vi "Actor Core.vi"(8 "error in":errorcluster, 11 "SpectrometerUI in":refnum<class "SpectrometerUI.lvclass">) -> (0 "error out":errorcluster, 3 "Actor out":refnum<class "Actor.lvclass">)   [LabVIEW 2023, in "SpectrometerUI.lvlib" / "SpectrometerUI.lvclass"]
doc: "(<B>Filename</B>: Actor Framework.lvlib:Actor.lvclass:Actor Core.vi)\n\nReceives messages to the actor, reacts to them, and initiates any error handling that may shut the actor down.\n\nDescendant classes may override this VI to append parallel tasks for the actor to complete while it handles messages. Overrides use the Call Parent Class Method node."
uses:
  SpectrometerUI.lvclass
  C:/Program Files/National Instruments/LabVIEW 2023/vi.lib/ActorFramework/Actor/Actor.lvclass
  <vilib>/ActorFramework/Actor/Actor.lvclass
  <vilib>/ActorFramework/Message Enqueuer/Message Enqueuer.lvclass
  typedefs/SpectroData.ctl
  ConcreteClasses/ConcreteInstrumentClasses/SpectrometerClasses/Spectrometer_HRS_LV/HRS_Spectrometer/HRS_Spectrometer/HRS_Spectrometer.lvclass
  <vilib>/ActorFramework/Actor/Actor.lvclass/Actor.ctl
  <vilib>/ActorFramework/Message Enqueuer/Message Enqueuer.lvclass/Message Enqueuer.ctl
  SpectrometerUI.lvclass/SpectrometerUI.ctl
  Interfaces/InitDeinitInterface/InitDeinit Messages/Init Msg/Init Msg.lvclass/Init Msg.ctl
  Interfaces/AbstractInstrumentClasses/Spectrometers_LV/Spectrometer Messages/GoToWavelength Msg/GoToWavelength Msg.lvclass/GoToWavelength Msg.ctl
  Interfaces/AbstractInstrumentClasses/Spectrometers_LV/Spectrometer Messages/SetMirror Msg/SetMirror Msg.lvclass/SetMirror Msg.ctl
  Interfaces/AbstractInstrumentClasses/Spectrometers_LV/Spectrometer Messages/SetSlitwidth Msg/SetSlitwidth Msg.lvclass/SetSlitwidth Msg.ctl
  Interfaces/AbstractInstrumentClasses/Spectrometers_LV/Spectrometer Messages/ChangeGrating Msg/ChangeGrating Msg.lvclass/ChangeGrating Msg.ctl
  <vilib>/ActorFramework/Message Enqueuer/Init from Existing Queue.vi
  <vilib>/ActorFramework/Message Enqueuer/Enqueue.vi
  Interfaces/InitDeinitInterface/InitDeinit Messages/DeInit Msg/DeInit Msg.lvclass
  C:/Program Files/National Instruments/LabVIEW 2023/vi.lib/ActorFramework/Message/Message.lvclass
  Interfaces/InitDeinitInterface/InitDeinit Messages/Init Msg/Init Msg.lvclass
  Interfaces/AbstractInstrumentClasses/Spectrometers_LV/Spectrometer Messages/GoToWavelength Msg/GoToWavelength Msg.lvclass
  Interfaces/AbstractInstrumentClasses/Spectrometers_LV/Spectrometer Messages/SetMirror Msg/SetMirror Msg.lvclass
  <vilib>/ActorFramework/Stop Msg/Stop Msg.lvclass
  Interfaces/AbstractInstrumentClasses/Spectrometers_LV/Spectrometer Messages/SetSlitwidth Msg/SetSlitwidth Msg.lvclass
  Interfaces/AbstractInstrumentClasses/Spectrometers_LV/Spectrometer Messages/ChangeGrating Msg/ChangeGrating Msg.lvclass
  <vilib>/ActorFramework/Message Priority Queue/Priority Enqueue.vi
  SpectrometerUI.lvlib
  typedefs/typedefs.lvlib
panel:
  out "Self Enqueuer":refnum<class "Message Enqueuer.lvclass">
  in  "stop":bool
  in  "Set FrEnt Slitwidth":bool
  in  "Front Entrance":dbl
  in  "Set SidEnt Slitwidth":bool
  in  "Side Entrance":dbl
  in  "Set FrExSlitwidth":bool
  in  "Front Exit":dbl
  in  "Exit":enum16{"FRONT", "SIDE"}(ring)
  in  "Entrance":enum16{"FRONT", "SIDE"}(ring)
  in  "SpectroCluster":T1
  out "HRS Enqueuer":refnum<class "Message Enqueuer.lvclass">
  in  "Set Grating":bool
  in  "Grating":u8=1 min=1 max=3
  in  "Set Wavelength":bool
  in  "Wavelength":dbl
  in  "Set SidExSlitwidth":bool
  in  "Side Exit":dbl
  in  "Connect":bool
  in  "VISA resource name":refnum<visa-resource-name>
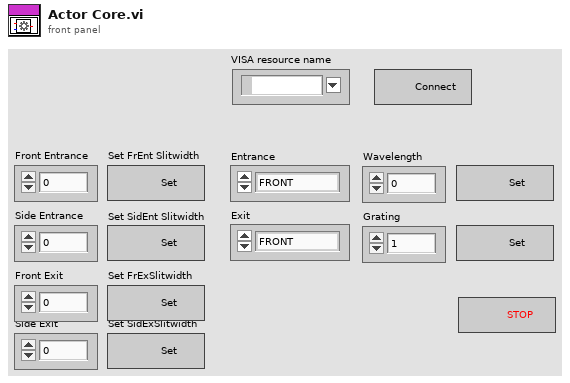
[diagram p1: front panel]
types:
  T1 = typedef "typedefs.lvlib/SpectroData.ctl" = cluster{"Wavelength":dbl, "Grating":u8, "Entrance ":enum16{"FRONT", "SIDE"}, "Exit ":enum16{"FRONT", "SIDE"}, "Entrance Front Slitwidth":u16, "Entrance Side Slitwidth":u16, "Exit Front Slitwidth":u16, "Exit Side Slitwidth":u16}
  T2 = enum16{"Front Entrance", "Side Entrance", "Front Exit", "Side Exit"}
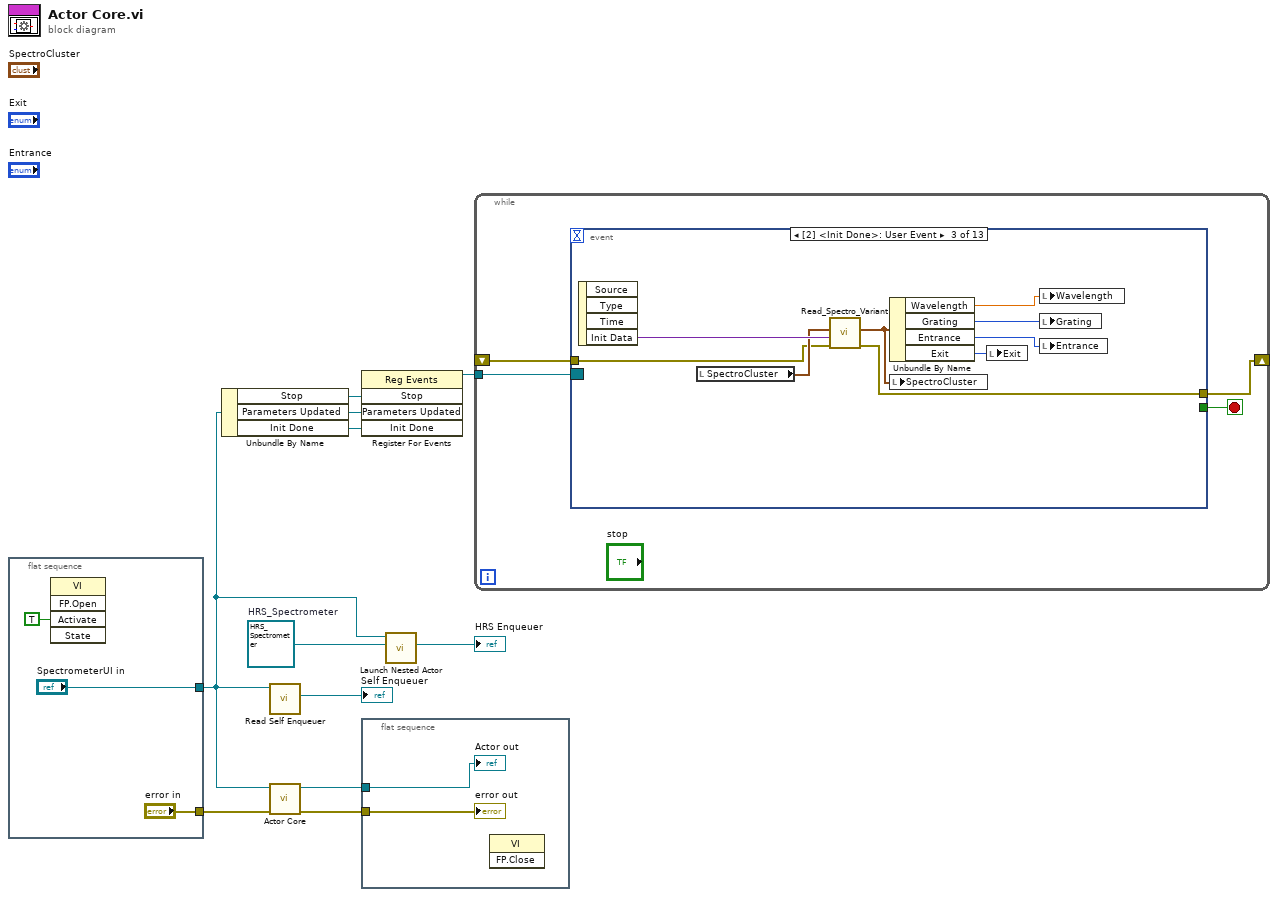
[diagram p0: block diagram]
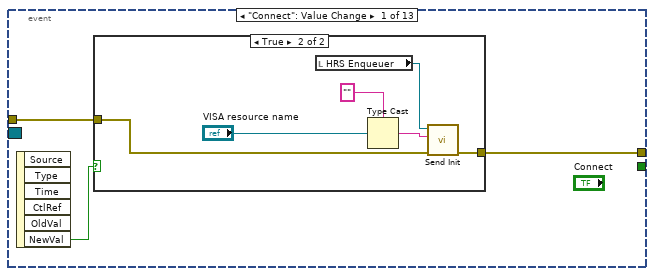
[diagram p2: hidden frame]
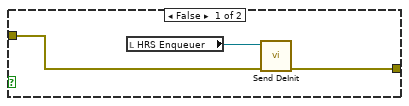
[diagram p3: hidden frame]
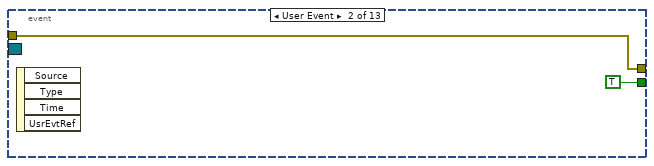
[diagram p4: hidden frame]
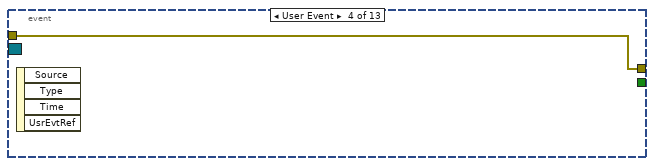
[diagram p5: hidden frame]
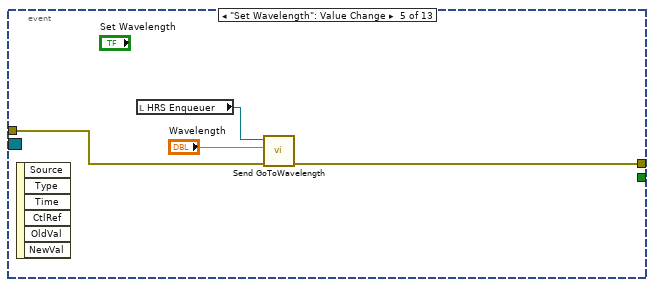
[diagram p6: hidden frame]
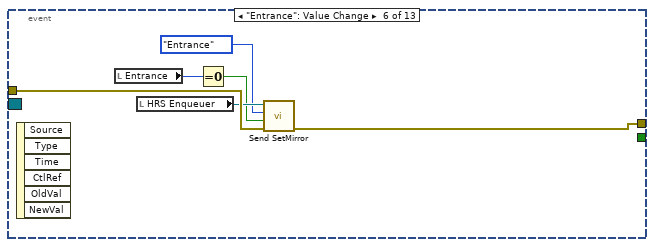
[diagram p7: hidden frame]
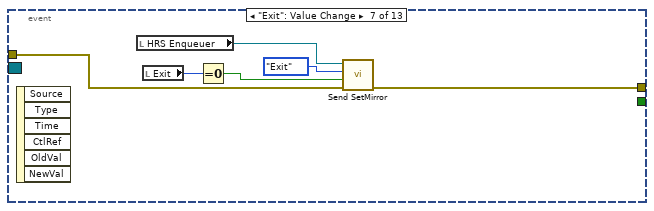
[diagram p8: hidden frame]
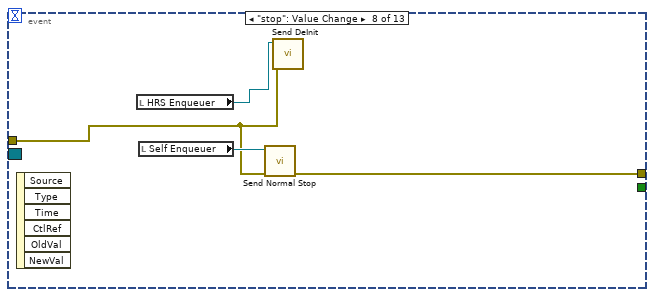
[diagram p9: hidden frame]
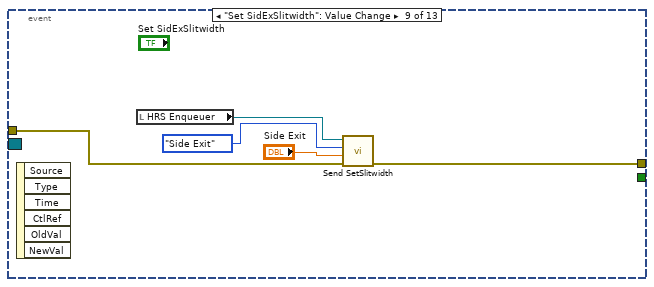
[diagram p10: hidden frame]
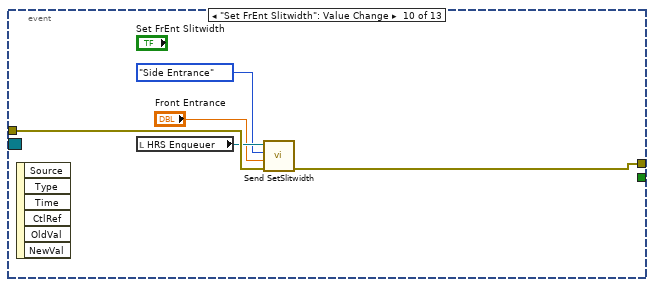
[diagram p11: hidden frame]
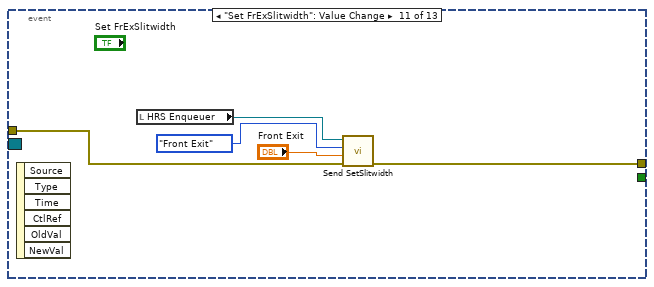
[diagram p12: hidden frame]
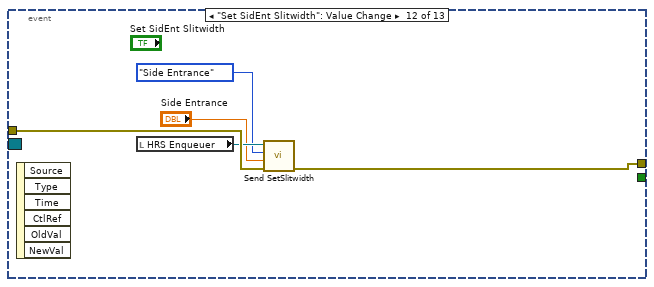
[diagram p13: hidden frame]
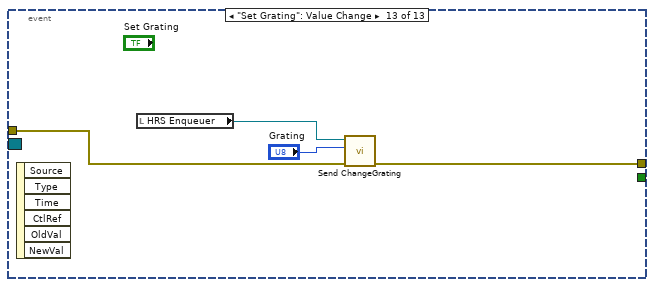
[diagram p14: hidden frame]
diagram:
  w9 = refnum<class "HRS_Spectrometer.lvclass"> refnum  # HRS_Spectrometer
  n1 = flat-sequence {
    tunnel: ["error in"] -> w11
    tunnel: ["SpectrometerUI in"] -> w2
    frame #0 {
      n2 = invoke class="VI" method="FP.Open"("Activate"=TRUE ("Activate?")) -> ()  [unwired: 4 in, 5 out]
    }
  }
  n3 = Unbundle By Name(w2) -> ("Stop"=w7:refnum<user-event>, "Parameters Updated"=w6:refnum<user-event>, "Init Done"=w5:refnum<user-event>)
  n4 = call <vilib>:"Read Self Enqueuer.vi"("Actor"=w2) -> ("Self Enqueuer"=→"Self Enqueuer":refnum<class "Message Enqueuer.lvclass">)  [unwired: 10 in]
  n5 = call-parent "Actor Core.vi"("error in"=w11, "Actor in"=w2) -> ("error out"=w3:errorcluster, "Actor out"=w4:refnum<class "Actor.lvclass">)  [unwired: 8 in]
  n6 = register-events(w7, w6, w5) -> (reference out=w8:refnum<event-registration>)  [unwired: 2 in, 1 out]
  n7 = flat-sequence {
    tunnel: w4 -> [w16]
    tunnel: w3 -> [w15]
    frame #0 {
      n8 = invoke class="VI" method="FP.Close"() -> ()  [unwired: 3 in, 3 out]
      "error out" <- w15
      "Actor out" <- w16
    }
  }
  n9 = call <vilib>:"Launch Nested Actor.vi"("Nested Actor"=w9, "Caller Actor in"=w2) -> ("Nested Actor's Enqueuer"=→"HRS Enqueuer":refnum<class "Message Enqueuer.lvclass">)  [unwired: 7 in, 2 out]
  n10 = while {
    shift-right: [w19] -> _
    shift-left: _ -> [w20]
    tunnel: w8 -> [w18]
    stop <- w17 stop-if-true
    n11 = event shown="[2] <Init Done>: User Event" {
      selector: w18 -> [_ _ _ _ _ _ _ _ _ _ _ _ _]
      dyn-events: _ -> [_ _ _ _ _ _ _ _ _ _ _ _ _]
      timeout: _ -> [_ _ _ _ _ _ _ _ _ _ _ _ _]
      tunnel: w20 -> [w23 w33 w41 w44 w47 w54 w60 w61 w68 w74 w79 w84 w88]
      tunnel: [w22 w33 w40 w44 w46 w53 w59 w63 w67 w73 w78 w83 w87] -> w19
      tunnel: [_ TRUE _ _ _ _ _ _ _ _ _ _ _] -> w17
      event "Connect": Value Change {
        n12 = event-data() -> ("NewVal"=w21:bool)  [unwired: 1 in, 5 out]
        n13 = case shown="True" w21 {
          tunnel: w23 -> [w26 w29]
          tunnel: [w25 w28] -> w22
          frame False {
            n14 = local read "HRS Enqueuer"() -> (w24:refnum<class "Message Enqueuer.lvclass">)
            n15 = call "Send DeInit.vi"("error in (no error)"=w26, "Message Enqueuer"=w24) -> ("error out"=w25:errorcluster)  [unwired: 8 in, 1 out]
          }
          frame True {
            n16 = local read "HRS Enqueuer"() -> (w27:refnum<class "Message Enqueuer.lvclass">)
            n17 = Type Cast(type="" ("Address"), x="VISA resource name") -> (*(type *) &x=w30:string)
            n18 = call "Send Init.vi"("error in (no error)"=w29, "Address"=w30, "Message Enqueuer"=w27) -> ("error out"=w28:errorcluster)  [unwired: 7 in, 1 out]
          }
        }
      }
      event User Event {
        n19 = event-data() -> ()  [unwired: 1 in, 4 out]
      }
      event User Event {
        n20 = event-data() -> ("Init Data"=w43:variant)  [unwired: 1 in, 3 out]
        n21 = local read "SpectroCluster"() -> (w42:T1)
        n22 = call "Read_Spectro_Variant.vi"("error in (no error)"=w41, "Variant"=w43, "SpectroCluster"=w42) -> ("error out"=w40:errorcluster, "SpectroCluster"=w39:T1)  [unwired: 7 in]
        n23 = Unbundle By Name(w39) -> ("Wavelength"=w37:dbl, "Grating"=w38:u8, "Entrance"=w36:enum16{"FRONT", "SIDE"}, "Exit"=w35:enum16{"FRONT", "SIDE"})
        n24 = local write "SpectroCluster"(w39) -> ()
        n25 = local write "Exit"(w35) -> ()
        n26 = local write "Wavelength"(w37) -> ()
        n27 = local write "Grating"(w38) -> ()
        n28 = local write "Entrance"(w36) -> ()
      }
      event User Event {
        n29 = event-data() -> ()  [unwired: 1 in, 4 out]
      }
      event "Set Wavelength": Value Change {
        n30 = event-data() -> ()  [unwired: 1 in, 6 out]
        n31 = local read "HRS Enqueuer"() -> (w45:refnum<class "Message Enqueuer.lvclass">)
        n32 = call "Send GoToWavelength.vi"("error in (no error)"=w47, "Wavelength"="Wavelength", "Message Enqueuer"=w45) -> ("error out"=w46:errorcluster)  [unwired: 7 in, 1 out]
      }
      event "Entrance": Value Change {
        n33 = event-data() -> ()  [unwired: 1 in, 6 out]
        n34 = local read "Entrance"() -> (w50:enum16{"FRONT", "SIDE"})
        n35 = local read "HRS Enqueuer"() -> (w52:refnum<class "Message Enqueuer.lvclass">)
        n36 = Equal To 0?(x=w50) -> (x = 0?=w49:bool)
        n37 = call "Send SetMirror.vi"("error in (no error)"=w54, "Front/Side"=w49, "Mirror"=enum16{"Entrance", "Exit"}."Entrance", "Message Enqueuer"=w52) -> ("error out"=w53:errorcluster)  [unwired: 6 in, 1 out]
      }
      event "Exit": Value Change {
        n38 = event-data() -> ()  [unwired: 1 in, 6 out]
        n39 = local read "HRS Enqueuer"() -> (w58:refnum<class "Message Enqueuer.lvclass">)
        n40 = local read "Exit"() -> (w56:enum16{"FRONT", "SIDE"})
        n41 = Equal To 0?(x=w56) -> (x = 0?=w55:bool)
        n42 = call "Send SetMirror.vi"("error in (no error)"=w60, "Front/Side"=w55, "Mirror"=enum16{"Entrance", "Exit"}."Exit", "Message Enqueuer"=w58) -> ("error out"=w59:errorcluster)  [unwired: 6 in, 1 out]
      }
      event "stop": Value Change {
        n43 = event-data() -> ()  [unwired: 1 in, 6 out]
        n44 = local read "HRS Enqueuer"() -> (w62:refnum<class "Message Enqueuer.lvclass">)
        n45 = local read "Self Enqueuer"() -> (w64:refnum<class "Message Enqueuer.lvclass">)
        n46 = call <vilib>:"Send Normal Stop.vi"("error in (no error)"=w61, "Message Enqueuer"=w64) -> ("error out"=w63:errorcluster)  [unwired: 9 in]
        n47 = call "Send DeInit.vi"("error in (no error)"=w61, "Message Enqueuer"=w62) -> ()  [unwired: 8 in, 2 out]
      }
      event "Set SidExSlitwidth": Value Change {
        n48 = event-data() -> ()  [unwired: 1 in, 6 out]
        n49 = local read "HRS Enqueuer"() -> (w66:refnum<class "Message Enqueuer.lvclass">)
        n50 = call "Send SetSlitwidth.vi"("error in (no error)"=w68, "Slitwidth"="Side Exit", "Slit"=T2."Side Exit", "Message Enqueuer"=w66) -> ("error out"=w67:errorcluster)  [unwired: 6 in, 1 out]
      }
      event "Set FrEnt Slitwidth": Value Change {
        n51 = event-data() -> ()  [unwired: 1 in, 6 out]
        n52 = local read "HRS Enqueuer"() -> (w72:refnum<class "Message Enqueuer.lvclass">)
        n53 = call "Send SetSlitwidth.vi"("error in (no error)"=w74, "Slitwidth"="Front Entrance", "Slit"=T2."Side Entrance", "Message Enqueuer"=w72) -> ("error out"=w73:errorcluster)  [unwired: 6 in, 1 out]
      }
      event "Set FrExSlitwidth": Value Change {
        n54 = event-data() -> ()  [unwired: 1 in, 6 out]
        n55 = local read "HRS Enqueuer"() -> (w77:refnum<class "Message Enqueuer.lvclass">)
        n56 = call "Send SetSlitwidth.vi"("error in (no error)"=w79, "Slitwidth"="Front Exit", "Slit"=T2."Front Exit", "Message Enqueuer"=w77) -> ("error out"=w78:errorcluster)  [unwired: 6 in, 1 out]
      }
      event "Set SidEnt Slitwidth": Value Change {
        n57 = event-data() -> ()  [unwired: 1 in, 6 out]
        n58 = local read "HRS Enqueuer"() -> (w82:refnum<class "Message Enqueuer.lvclass">)
        n59 = call "Send SetSlitwidth.vi"("error in (no error)"=w84, "Slitwidth"="Side Entrance", "Slit"=T2."Side Entrance", "Message Enqueuer"=w82) -> ("error out"=w83:errorcluster)  [unwired: 6 in, 1 out]
      }
      event "Set Grating": Value Change {
        n60 = event-data() -> ()  [unwired: 1 in, 6 out]
        n61 = local read "HRS Enqueuer"() -> (w85:refnum<class "Message Enqueuer.lvclass">)
        n62 = call "Send ChangeGrating.vi"("error in (no error)"=w88, "Grating"="Grating", "Message Enqueuer"=w85) -> ("error out"=w87:errorcluster)  [unwired: 7 in, 1 out]
      }
    }
  }
